vi "Example_Fitting.vi"() -> ()   [LabVIEW 2016]
panel:
  out "Gaussian":dbl[][](graph)
  out "Lorentzian":dbl[][](graph)
  out "Intensity Graph":dbl[][](graph)
  in  "a":dbl[](array[numeric])
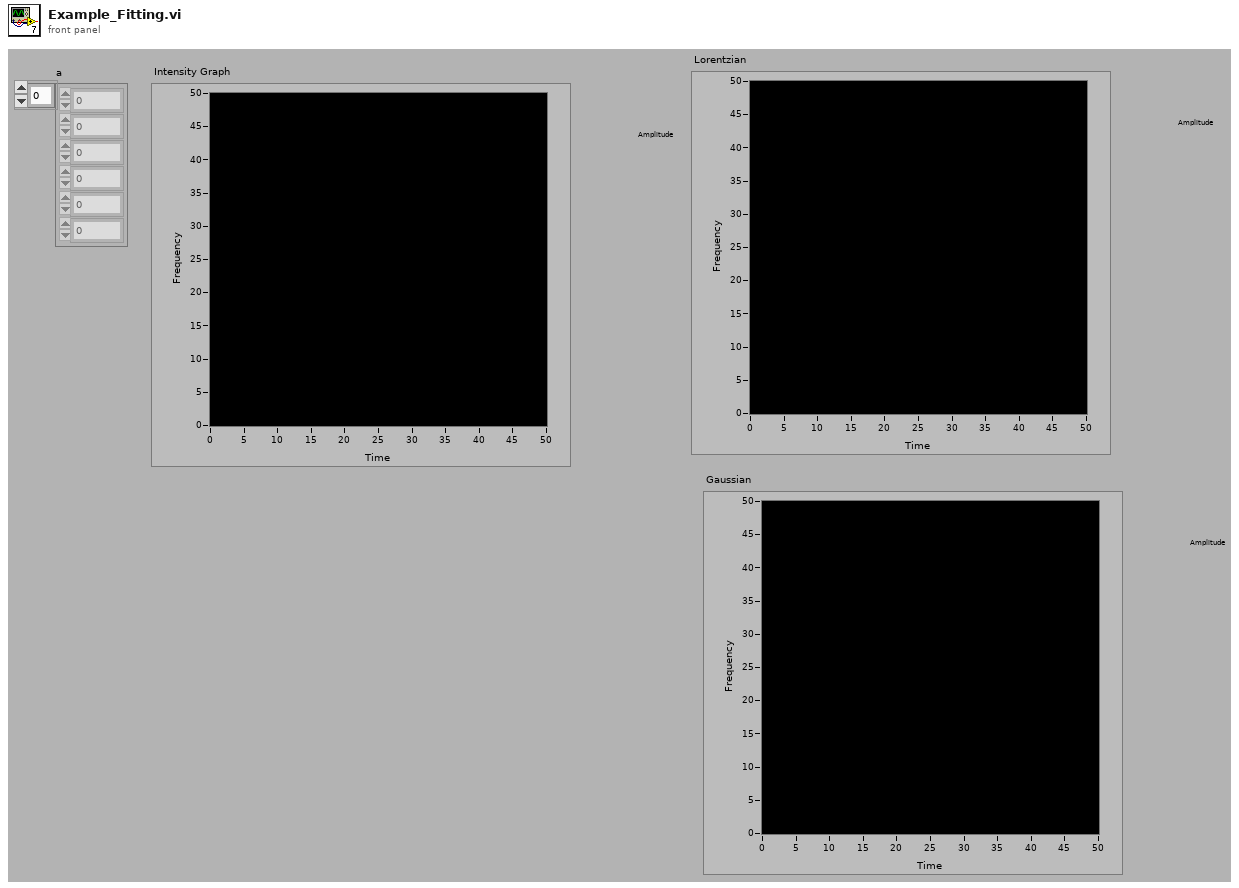
[diagram p1: front panel]
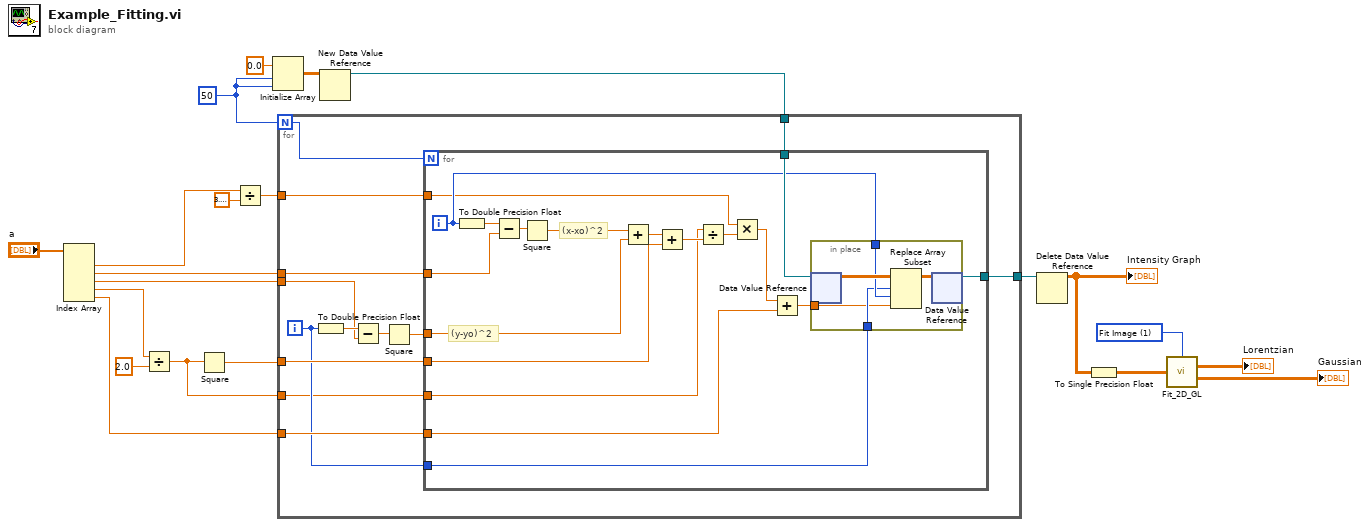
[diagram p0: block diagram]
diagram:
  w1 = u16 1 items=["Read Fit Data", "Fit Image"] ("Action")
  w6 = 50
  n1 = Index Array(array="a") -> (element #1=w12:dbl, element #2=w20:dbl, element #3=w19:dbl, element #4=w10:dbl, element #5=w14:dbl)  [unwired: 5 in]
  n2 = Divide(x=w10, y=2.0) -> (x/y=w7:dbl)
  n3 = Square(x=w7) -> (x^2=w8:dbl)
  n4 = Divide(x=w12, y=3.141592653589793) -> (x/y=w11:dbl)
  n5 = Initialize Array(0.0 ("element"), w6, w6) -> (w17:dbl[][])
  n6 = New Data Value Reference(data value=w17) -> (data value reference=w16:refnum<data-value>)  [unwired: 1 in, 1 out]
  n7 = for {
    N: w6 -> [w34]
    tunnel: w11 -> [w33]
    tunnel: w20 -> [w32]
    tunnel: w19 -> [w29]
    tunnel: w14 -> [w31]
    tunnel: w8 -> [w26]
    tunnel: w16 -> [w25]
    tunnel: [w23] -> w15
    tunnel: w7 -> [w22]
    i -> [w24]
    n8 = To Double Precision Float(number=w24) -> (double precision float=w30:dbl)
    n9 = Subtract(x=w30, y=w29) -> (x-y=w28:dbl)
    n10 = Square(x=w28) -> (x^2=w27:dbl)
    n11 = for {
      N: w34 -> [_]
      tunnel: w33 -> [w38]
      tunnel: w32 -> [w51]
      tunnel: w31 -> [w36]
      tunnel: w27 -> [w41]
      tunnel: w26 -> [w43]
      tunnel: w25 -> [w49]
      tunnel: w24 -> [w47]
      tunnel: [w46] -> w23
      tunnel: w22 -> [w40]
      i -> [w48]
      # "(y-yo)^2"
      # "(x-xo)^2"
      n12 = To Double Precision Float(number=w48) -> (double precision float=w52:dbl)
      n13 = Subtract(x=w52, y=w51) -> (x-y=w50:dbl)
      n14 = Square(x=w50) -> (x^2=w42:dbl)
      n15 = Add(x=w42, y=w41) -> (x+y=w45:dbl)
      n16 = Add(x=w45, y=w43) -> (x+y=w44:dbl)
      n17 = Divide(x=w40, y=w44) -> (x/y=w39:dbl)
      n18 = Multiply(x=w38, y=w39) -> (x*y=w37:dbl)
      n19 = Add(x=w37, y=w36) -> (x+y=w35:dbl)
      n20 = in-place {
        in-place-border: w48 -> [w55]
        in-place-border: w47 -> [w54]
        in-place-border: w35 -> [w53]
        n21 = in-place-dvr #1(w49) -> (w57:dbl[][])  [unwired: 1 out]
        n22 = Replace Array Subset(array=w57, new element=w53, index (row)=w54, index (col)=w55) -> (w56:dbl[][])
        n23 = in-place-dvr #1(w56) -> (w46:refnum<data-value>)  [unwired: 1 out]
      }
    }
  }
  n24 = Delete Data Value Reference(data value reference=w15) -> (data value=w5:dbl[][])  [unwired: 1 in, 1 out]
  "Intensity Graph" <- w5
  n25 = To Single Precision Float(number=w5) -> (single precision float=w4:sgl[][])
  n26 = call "Fit_2D_GL.vi"("Action"=w1, "Image IN"=w4) -> ("Lorentzian Image"=→"Lorentzian":dbl[][], "Gaussian Image"=→"Gaussian":dbl[][])  [unwired: 9 in, 3 out]
